vi "RT_Main Queue.vi"(8 "error in":errorcluster) -> (0 "error out":errorcluster, 3 "Request Queue":refnum<queue>)   [LabVIEW 2018]
uses:
  Data Def/RT_Request Data.ctl
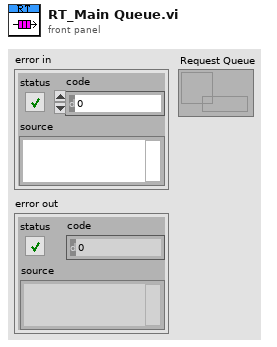
[diagram p1: front panel]
types:
  T1 = typedef "RT_Request Data.ctl" = cluster{"Connection ID":refnum<k5>, "Command":string, "Data":string}
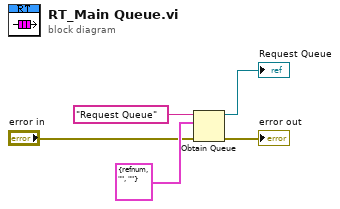
[diagram p0: block diagram]
diagram:
  n1 = Obtain Queue(name (unnamed)="Request Queue", element data type=T1 {"Connection ID"=refnum, "Command"="", "Data"=""} ("Request Data"), error in (no error)="error in") -> (queue out=→"Request Queue":refnum<queue>, error out=→"error out":errorcluster)  [unwired: 2 in, 1 out]
